vi "IsNULL.vi"(8 "error in (no error)":errorcluster, 11 "ptr":i64) -> (0 "error out":errorcluster)   [LabVIEW 2026, in "SDL3.lvlib" / "LV-Utilities.lvlib"]
doc: "<B>Summary</B>\nGenerate an error in case <B>ptr</B> is NULL (0)."
uses:
  LV-Utilities.lvlib
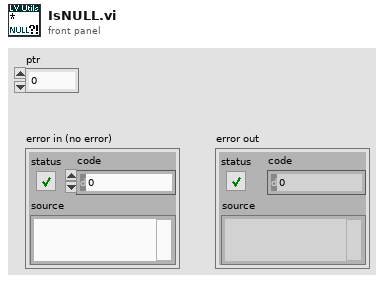
[diagram p1: front panel]
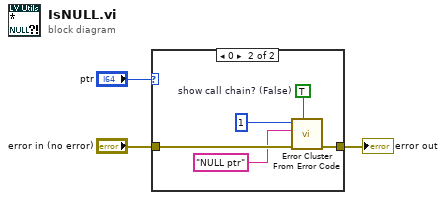
[diagram p0: block diagram]
diagram:
  n1 = case shown="0" "ptr" {
    tunnel: "error in (no error)" -> [w4 w9]
    tunnel: [w4 w8] -> w2
    frame Default {
    }
    frame 0 {
      w5 = TRUE  # show call chain? (False)
      n2 = call <vilib>:"Error Cluster From Error Code.vi"("show call chain? (False)"=w5, "error in (no error)"=w9, "error message (\"\")"="NULL ptr" ("error message (\"\")"), "error code (0)"=1) -> ("error out"=w8:errorcluster)  [unwired: 5 in]
    }
  }
  "error out" <- w2
